vi "DFD MRate Filtering (Wfm NChan).vi"(6 "zero phase? (T)":bool=TRUE, 7 "init? (F)":bool, 8 "error in (no error)":errorcluster, 10 "multirate filter":T1={"mMRate_Structure"=enum."IIR", "mMRate_Mode"=0, "mMRate_Factor"=-1, "mMRate_FIRParams"={"mMRate_FIR_H"=[], "mMRate_FIR_IsNyquist?"=FALSE, "mMRate_FIR_IsSymmetric?"=FALSE}, "mMRate_CICParams"={"mMRate_CIC_#Stage"=0, "mMRate_CIC_Lag"=0, "mMRate_CIC_Type"=enum."Lowpass"}, "mMRate_Order"=0, "mMRate_Version"="2.0", "mMRate_Comments"="", "mMRate_RationalFactor"={"mMRate_L"=-1, "mMRate_M"=-1}, "mMRate_Fs"=1.0, "mMRate_Quantized?"=FALSE, "mMRate_QFilterGain"=1.0, "mMRate_CoefWl"=16, "mMRate_Scaling"={"mMRate_ScaleByPowerOf2?"=FALSE, "mMRate_ScaleType"=enum."No Norm"}, "mMRate_InputWl"=16, "mMRate_OutputWl"=16, "mMRate_OutputMode"=enum."Truncation", "mMRate_MultMode"=enum."Truncated", "mMRate_BitPruning"=FALSE, "mMRate_GainWl"=16, "mMRate_OutputFwl"=0, "mMRate_SumIwl"=0, "mMRate_InputIwl "=16, "mMRate_SumWl"=32, "mMRate_CoefIwl"=0} {"mMRate_SumWl" min=1 max=32 step=1; "mMRate_InputIwl" min=1 max=32 step=1; "mMRate_GainWl" min=1 max=32 step=1; "mMRate_OutputWl" min=1 max=32 step=1; "mMRate_InputWl" min=1 max=32 step=1; "mMRate_CoefWl" min=1 max=32 step=1; "mMRate_Mode" items=["Default"=-1, "No Rate Change"=0, "Interpolation"=1, "Decimation"=2, "Interpolated"=3, "Rational"=4]}, 11 "signal in":waveform(dbl)[](array[waveform])) -> (0 "error out":errorcluster, 3 "signal out":waveform(dbl)[](array[waveform]))   [LabVIEW 2017, in "NI_DigFilterLicensed.lvlib"]
doc: "Filters a signal continuously with a multirate filter. Wire data to the <B>signal in</B> input to determine the polymorphic instance to use or manually select the instance."
uses:
  <vilib>/addons/Digital Filter Design/NI_DigFilterLicensed.lvlib
  <vilib>/addons/Digital Filter Design/_Objects.llb/DFD Multirate Filter Obj.ctl
  <vilib>/addons/Digital Filter Design/_Objects.llb/DFD Multirate Mode.ctl
  <vilib>/addons/Digital Filter Design/_Objects.llb/DFD Coef Norm Type.ctl
  <vilib>/addons/Digital Filter Design/_Objects.llb/DFD Round-off Mode.ctl
  <vilib>/addons/Digital Filter Design/_Objects.llb/DFD FXP MRate Multiply Mode.ctl
  <vilib>/addons/Digital Filter Design/NI_DigFilter_Process.lvlib
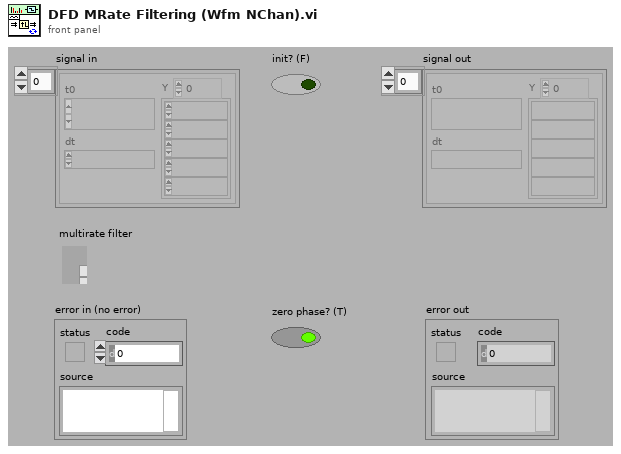
[diagram p1: front panel]
types:
  T1 = typedef "NI_DigFilterLicensed.lvlib/DFD Multirate Filter Obj.ctl" = cluster{"mMRate_Structure":enum16{"CIC", "FIR", "IIR", "Lattice"}, "mMRate_Mode":T2, "mMRate_Factor":i32, "mMRate_FIRParams":cluster{"mMRate_FIR_H":dbl[], "mMRate_FIR_IsNyquist?":bool, "mMRate_FIR_IsSymmetric?":bool}, "mMRate_CICParams":cluster{"mMRate_CIC_#Stage":i32, "mMRate_CIC_Lag":i32, "mMRate_CIC_Type":enum16{"Lowpass", "Highpass"}}, "mMRate_Order":i32, "mMRate_Version":string, "mMRate_Comments":string, "mMRate_RationalFactor":cluster{"mMRate_L":i32, "mMRate_M":i32}, "mMRate_Fs":dbl, "mMRate_Quantized?":bool, "mMRate_QFilterGain":dbl, "mMRate_CoefWl":i16, "mMRate_Scaling":cluster{"mMRate_ScaleByPowerOf2?":bool, "mMRate_ScaleType":T3}, "mMRate_InputWl":i16, "mMRate_OutputWl":i16, "mMRate_OutputMode":T4, "mMRate_MultMode":T5, "mMRate_BitPruning":bool, "mMRate_GainWl":i16, "mMRate_OutputFwl":i16, "mMRate_SumIwl":i16, "mMRate_InputIwl ":i16, "mMRate_SumWl":i16, "mMRate_CoefIwl":i16}
  T2 = typedef "NI_DigFilterLicensed.lvlib/DFD Multirate Mode.ctl" = i16
  T3 = typedef "NI_DigFilterLicensed.lvlib/DFD Coef Norm Type.ctl" = enum16{"No Norm", "Time Domain 1-Norm", "Time Domain 2-Norm", "Time Domain Inf-Norm"}
  T4 = typedef "NI_DigFilterLicensed.lvlib/DFD Round-off Mode.ctl" = enum16{"Nearest", "Truncation"}
  T5 = typedef "NI_DigFilterLicensed.lvlib/DFD FXP MRate Multiply Mode.ctl" = enum16{"Truncated", "Full"}
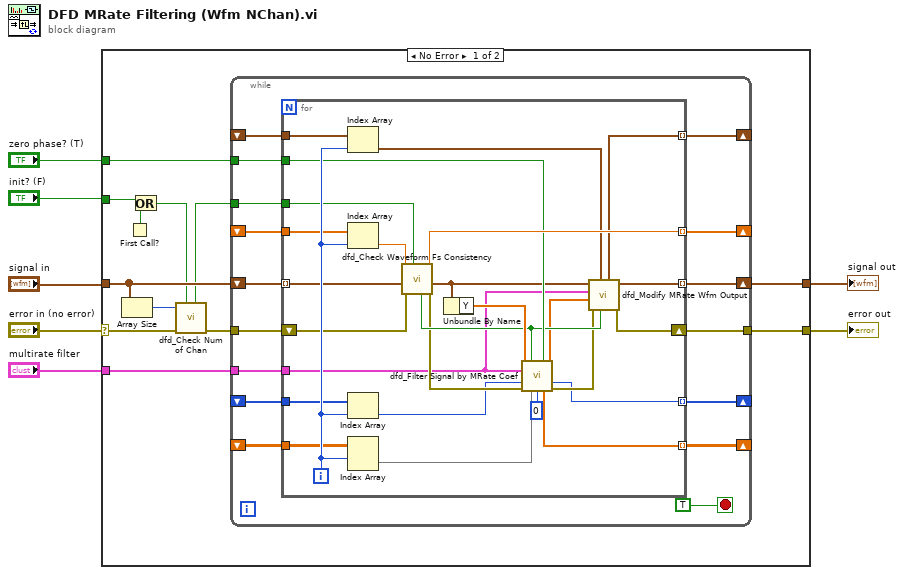
[diagram p0: block diagram]
diagram:
  n1 = case shown="No Error" "error in (no error)" {
    selector: "error in (no error)" -> [w12 w63]
    tunnel: [w19 w63] -> w4
    tunnel: "signal in" -> [w15 w64]
    tunnel: [w9 w64] -> w6
    tunnel: "init? (F)" -> [w16 _]
    tunnel: "zero phase? (T)" -> [w18 _]
    tunnel: "multirate filter" -> [w8 _]
    frame No Error {
      n2 = Array Size(array=w15) -> (size(s)=w14:i32)
      n3 = First Call?() -> (First Call?: T/F=w17:bool)
      n4 = Or(x=w16, y=w17) -> (x .or. y?=w13:bool)
      n5 = call <vilib>:"dfd_Check Num of Chan.vi"("init in"=w13, "error in (no error)"=w12, "#ch in"=w14) -> ("error out"=w10:errorcluster, "init out"=w11:bool)  [unwired: 7 out]
      n6 = while {
        shift-right: [w20] -> _
        shift-left: _ -> [w30]
        tunnel: [w29] -> w19
        tunnel: w11 -> [w25]
        shift-right: [w24] -> _
        shift-left: _ -> [w33]
        shift-right: [w26] -> _
        shift-left: _ -> [w32]
        tunnel: w18 -> [w28]
        shift-right: [w21] -> _
        shift-left: _ -> [w31]
        tunnel: w10 -> [w27]
        shift-right: [w23] -> w9
        shift-left: w15 -> [w35]
        tunnel: w8 -> [w22]
        stop <- TRUE stop-if-true
        n7 = for {
          tunnel: w35 -> [w61] mode=indexing
          tunnel: w30 -> [w38]
          tunnel: w33 -> [w51]
          shift-right: [w44] -> w29
          shift-left: w27 -> [w47]
          tunnel: w32 -> [w60]
          tunnel: w31 -> [w42]
          tunnel: w28 -> [w55]
          tunnel: [w58] -> w26 mode=indexing
          tunnel: w25 -> [w57]
          tunnel: [w49] -> w24 mode=indexing
          tunnel: [w48] -> w23 mode=indexing
          tunnel: w22 -> [w43]
          tunnel: [w41] -> w21 mode=indexing
          tunnel: [w39] -> w20 mode=indexing
          i -> [w62]
          n8 = Index Array(array=w51, index=w62) -> (element=w50:timestamp)
          n9 = Index Array(array=w60, index=w62) -> (element=w59:dbl)
          n10 = Index Array(array=w42, index=w62) -> (element=w40:i32)
          n11 = Index Array(array=w38, index (row)=w62) -> (element=w37:dbl[])  [unwired: 1 in]
          n12 = call <vilib>:"dfd_Check Waveform Fs Consistency.vi"("init in"=w57, "error in (no error)"=w47, "signal in"=w61, "dt in"=w59) -> ("error out"=w46:errorcluster, "signal out"=w52:waveform(dbl), "dt out"=w58:dbl, "init out"=w54:bool)  [unwired: 4 out]
          n13 = Unbundle By Name(w52) -> ("Y"=w56:dbl[])
          n14 = call <vilib>:"dfd_Filter Signal by MRate Coef.vi"("signal in"=w56, "initH?"=w54, "zeroPhaseH?"=w55, "multirate filter"=w43, "skipPoint In"=w40, "error in (no error)"=w46, "state in"=w37, "outputPhase"=0) -> ("signal out"=w53:dbl[], "skipPoint Out"=w41:i32, "state out"=w39:dbl[], "error out"=w45:errorcluster)  [unwired: 4 out]
          n15 = call <vilib>:"dfd_Modify MRate Wfm Output.vi"("initH"=w54, "t0"=w50, "error in (no error)"=w45, "y"=w53, "multirate filter in"=w43, "x"=w52) -> ("error out"=w44:errorcluster, "y"=w48:waveform(dbl), "tf"=w49:timestamp)  [unwired: 3 out]
        }
      }
    }
    frame Error {
    }
  }
  "error out" <- w4
  "signal out" <- w6
